vi "dfd_CIC Integrater Simu.vi"(7 "stage":i32, 8 "acc in":T1[](array[typedef]), 9 "Decimation?":bool, 10 "Bit to cut":i32[](array[numeric]), 11 "x":T1) -> (0 "acc out":T1[](array[typedef]), 3 "y":T1)   [LabVIEW 2017, in "NI_DigFilter_FXP.lvlib"]
uses:
  <vilib>/addons/Digital Filter Design/NI_DigFilter_FXP.lvlib
  <vilib>/addons/Digital Filter Design/_Objects.llb/dfd_Integer I160.ctl
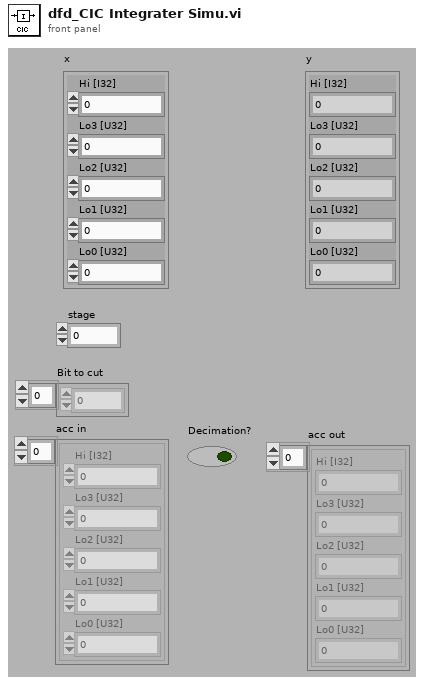
[diagram p1: front panel]
types:
  T1 = typedef "dfd_Integer I160.ctl" = cluster{"Hi [I32]":i32, "Lo3 [U32]":u32, "Lo2 [U32]":u32, "Lo1 [U32]":u32, "Lo0 [U32]":u32}
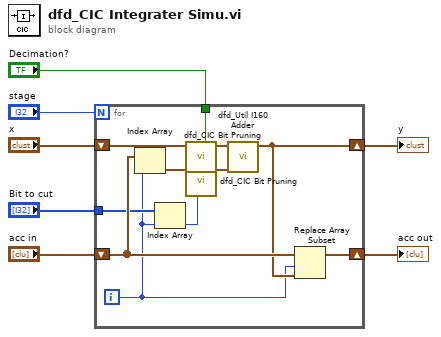
[diagram p0: block diagram]
diagram:
  n1 = for {
    N: "stage" -> [_]
    shift-right: [w18] -> w5
    shift-left: "acc in" -> [w17]
    shift-right: [w16] -> w6
    shift-left: "x" -> [w15]
    tunnel: "Bit to cut" -> [w11]
    tunnel: "Decimation?" -> [w8]
    i -> [w10]
    n2 = Index Array(array=w17, index=w10) -> (element=w13:T1)
    n3 = Index Array(array=w11, index=w10) -> (element=w9:i32)
    n4 = call <vilib>:"dfd_CIC Bit Pruning.vi"("cut?"=w8, "Bit to cut"=w9, "x"=w15) -> ("y"=w14:T1)  [unwired: 8 out]
    n5 = call <vilib>:"dfd_CIC Bit Pruning.vi"("cut?"=w8, "Bit to cut"=w9, "x"=w13) -> ("y"=w12:T1)  [unwired: 8 out]
    n6 = call <vilib>:"dfd_Util I160 Adder.vi"("y160"=w12, "x160"=w14) -> ("x+y160"=w16:T1)  [unwired: 9 out]
    n7 = Replace Array Subset(array=w17, new element=w16, index=w10) -> (w18:T1[])
  }
  "y" <- w6
  "acc out" <- w5
